vi "get Approach wfm.vi"(0 "reference in":refnum<class "Force Curve_tdms.lvclass">, 5 "error in (no error)":errorcluster) -> (14 "reference out":refnum<class "Force Curve_tdms.lvclass">, 16 "Samples Approach":i32, 19 "error out":errorcluster)   [LabVIEW 2019, in "Force Curve_tdms.lvclass"]
uses:
  Force Curve_tdms.lvclass
  private/Signal In.ctl
  <vilib>/Waveform/WDTOps.llb/WDT Get Waveform Subset DBL.vi
panel:
  out "actual duration (s)":dbl format="%0.2f"
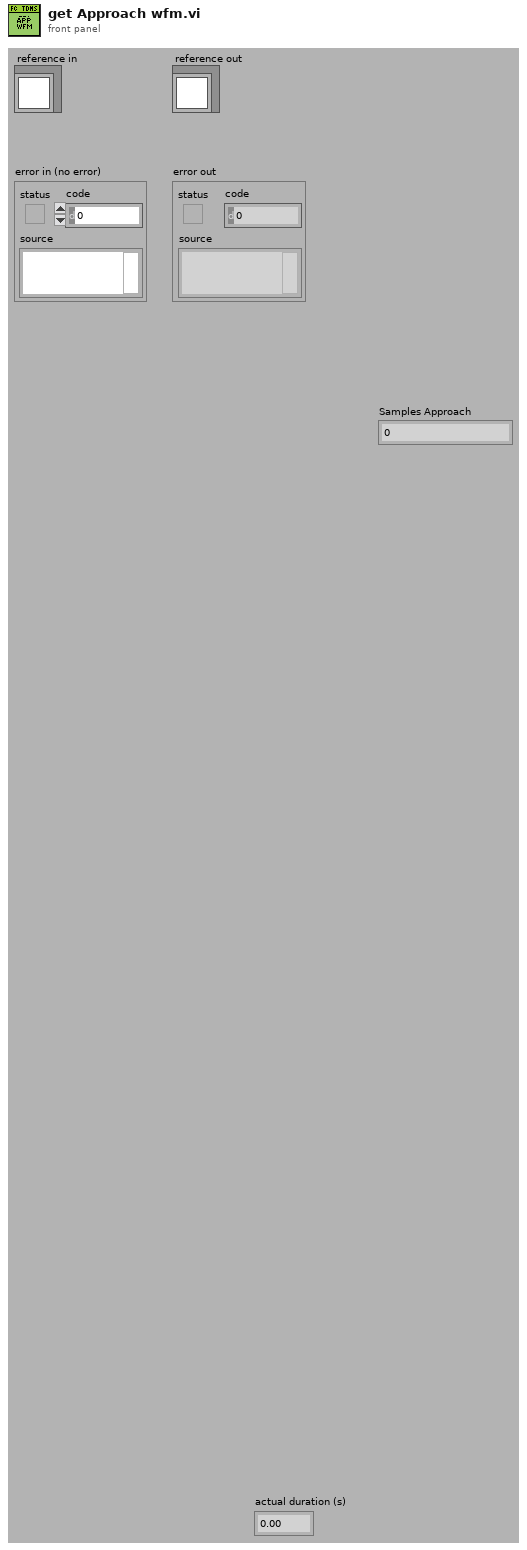
[diagram p1: front panel]
types:
  T1 = typedef "Force Curve_tdms.lvclass/Signal In.ctl" = enum16{"Deflection", "SensorIn", "MockOut", "ZstageOut"}
  T2 = typedef "Force Curve_tdms.lvclass/ObjectAttributesRef.ctl" = refnum<data-value>
  T3 = typedef "Force Curve_tdms.lvclass/ObjectAttributes.ctl" = cluster{"MyAttribute":dbl, "Processed data":waveform(dbl)[], "Fcurve Raw Metadata":T4, "Fcurve Metadata":T5, "Fcurve index":T6, "Tau Delay (ms)":dbl, "Contact Spread of dev":dbl, "Fcurve":T7}
  T4 = typedef "TDMS_DataHandler.lvclass/Fcurve Meta data.ctl" = cluster{"property names":string[], "property values":variant[]}
  T5 = typedef "Force Curve_tdms.lvclass/Fcurve Meta data analysis.ctl" = cluster{"dt (us)":dbl, "Dec Factor":dbl, "Z piezo Sensitivity (nm/V)":dbl, "K (N/m)":dbl, "Sp (V)":dbl, "Contact (ms)":dbl, "Zpos contact":dbl, "Vel_app (nm/s)":dbl, "Vel_ret (nm/s)":dbl, "deltaV (nm)":dbl, "Def_V0 (v)":dbl, "Decimating Factor":dbl}
  T6 = typedef "Force Curve_tdms.lvclass/Fcurve Index .ctl" = cluster{"Setpoint index":i32, "Max force index":i32, "Contact point index":i32, "Appoach indices":cluster{"Start":i32, "End":i32}, "Contact indices":cluster{"Start":i32, "End":i32}, "Retract indices":cluster{"Start":i32, "End":i32}}
  T7 = typedef "Force Curve_tdms.lvclass/Force Curve data.ctl" = cluster{"Approach":cluster{"X":dbl[], "Y":dbl[]}, "Contact":cluster{"X":dbl[], "Y":dbl[]}, "Retract":cluster{"X":dbl[], "Y":dbl[]}}
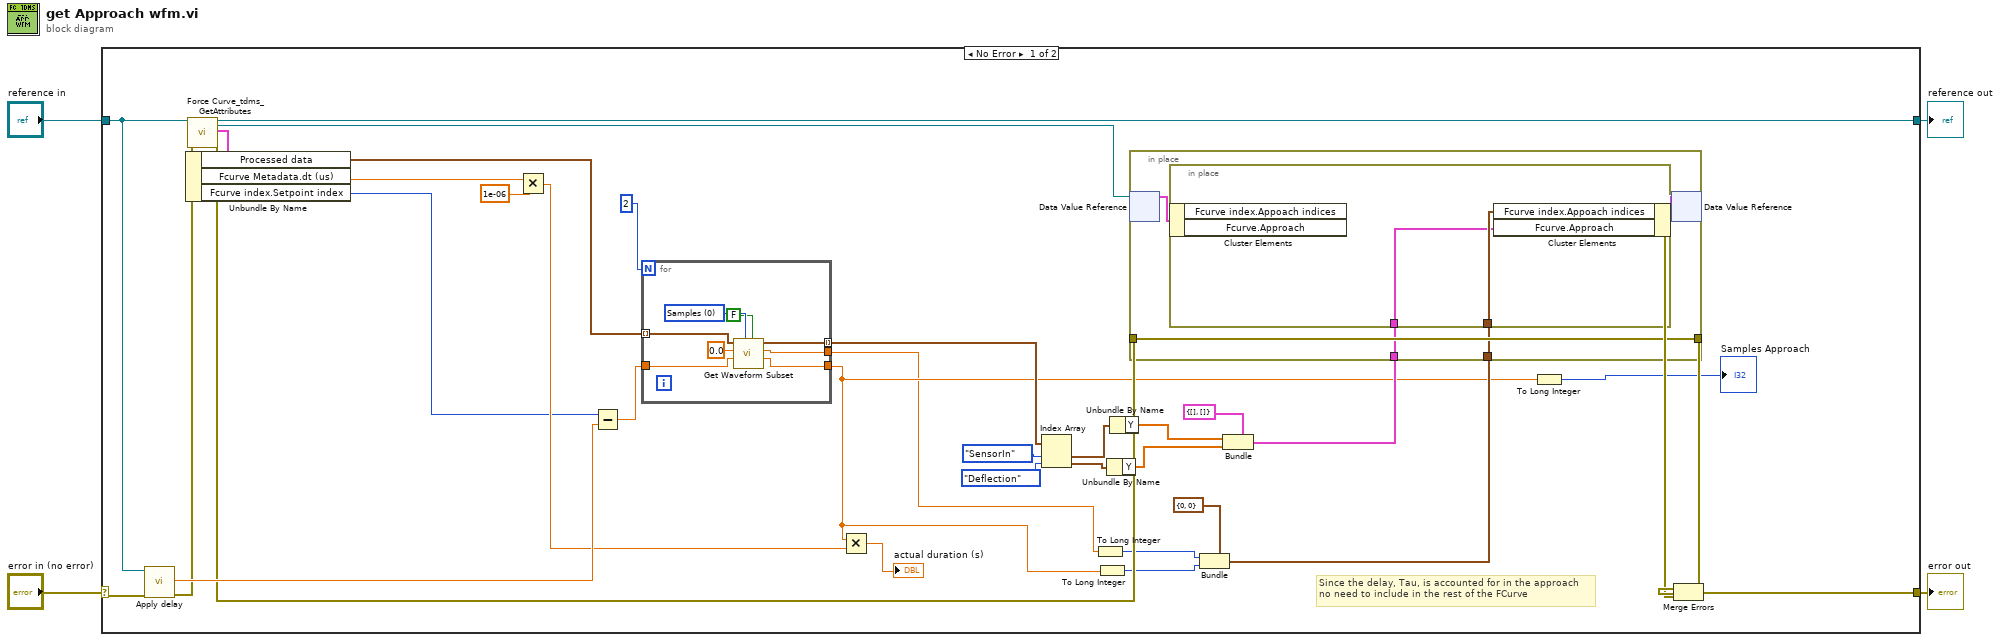
[diagram p0: block diagram]
diagram:
  n1 = case shown="No Error" "error in (no error)" {
    selector: "error in (no error)" -> [w14 w56]
    tunnel: [w39 w56] -> w3
    tunnel: [w38 w55] -> w1
    tunnel: "reference in" -> [w31 w55]
    frame No Error {
      # "Since the delay, Tau, is accounted for in the approach\nno need to include in the rest of the FCurve"
      n2 = call "Apply delay.vi"("reference in"=w31, "error in (no error)"=w14) -> ("# of samples"=w30:dbl, "error out"=w13:errorcluster)  [unwired: 15 in, 1 out]
      n3 = call "Force Curve_tdms_GetAttributes.vi"("reference in"=w31, "error in (no error)"=w13) -> ("reference out"=w38:refnum<class "Force Curve_tdms.lvclass">, "attributes ref"=w34:T2, "attributes"=w37:T3, "error out"=w12:errorcluster)  [unwired: 14 in]
      n4 = Unbundle By Name(w37) -> ("Processed data"=w32:waveform(dbl)[], "Fcurve Metadata.dt (us)"=w20:dbl, "Fcurve index.Setpoint index"=w15:i32)
      n5 = Multiply(x=w20, y=1e-06) -> (x*y=w18:dbl)
      n6 = Subtract(x=w15, y=w30) -> (x-y=w10:dbl)
      n7 = for {
        N: 2 -> [_]
        tunnel: w10 -> [w45]
        tunnel: [w44] -> w7
        tunnel: [w43] -> w27 mode=indexing
        tunnel: w32 -> [w42] mode=indexing
        tunnel: [w40] -> w6
        w47 = u16 0 items=["Samples", "Relative Time"] ("start/duration format")
        n8 = call-poly <vilib>:"Get Waveform Subset.vi"("open interval? (T)"=FALSE, "start/duration format"=w47, "duration"=w45, "start samples/time"=0.0, "waveform in"=w42) -> ("actual duration"=w44:dbl, "actual start samples/time"=w40:dbl, "waveform out"=w43:waveform(dbl))  [unwired: 1 in, 1 out]
      }
      n9 = Multiply(x=w7, y=w18) -> (x*y=→"actual duration (s)":dbl)
      n10 = Index Array(array=w27, index #1=Signal_In."SensorIn" ("Signal in"), index #2=Signal_In."Deflection" ("Signal in")) -> (element #1=w24:waveform(dbl), element #2=w23:waveform(dbl))
      n11 = To Long Integer(number=w6) -> (32bit integer=w5:i32)
      n12 = To Long Integer(number=w7) -> (32bit integer=w9:i32)
      n13 = Unbundle By Name(w23) -> ("Y"=w22:dbl[])
      n14 = Unbundle By Name(w24) -> ("Y"=w21:dbl[])
      n15 = Bundle(cluster=cluster{"Start":i32, "End":i32} {"Start"=0, "End"=0} ("Fcurve index.Appoach indices"), "Start"=w5, "End"=w9) -> (w8:cluster{"Start":i32, "End":i32})
      n16 = Bundle(cluster=cluster{"X":dbl[], "Y":dbl[]} {"X"=[], "Y"=[]} ("Fcurve.Approach"), "X"=w21, "Y"=w22) -> (w28:cluster{"X":dbl[], "Y":dbl[]})
      n17 = in-place {
        in-place-border: w12 -> [w50]
        in-place-border: [w50] -> w36
        in-place-border: w28 -> [w49]
        in-place-border: w8 -> [w48]
        n18 = in-place-dvr #1(w34) -> (w51:T3)  [unwired: 1 out]
        n19 = in-place {
          in-place-border: w49 -> [w53]
          in-place-border: w48 -> [w54]
          n20 = in-place-cluster #2(w51) -> ()  [unwired: 2 out]
          n21 = in-place-cluster #2("Fcurve index.Appoach indices"=w54, "Fcurve.Approach"=w53) -> (w52:T3)
        }
        n22 = in-place-dvr #1(w52) -> (w35:errorcluster)  [unwired: 1 out]
      }
      n23 = To Long Integer(number=w7) -> (32bit integer=→"Samples Approach":i32)
      n24 = Merge Errors(w36, w35) -> (w39:errorcluster)
    }
    frame Error {
    }
  }
  "error out" <- w3
  "reference out" <- w1
